vi "Prepend LBCB Number.vi"(1 "Prepended In":string[](array[string]), 2 "LBCB Number":T1, 3 "Names In":string[](array[string])) -> (0 "Prepended Out":string[](array[string]))   [LabVIEW 2013]
uses:
  Data Access Objects/Metadata/LBCB Number.ctl
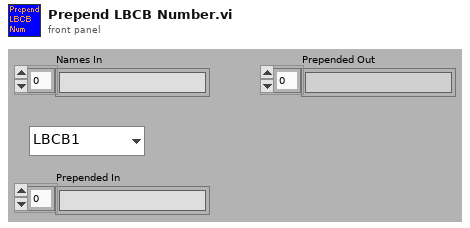
[diagram p1: front panel]
types:
  T1 = typedef "LBCB Number.ctl" = enum16{"LBCB1", "LBCB2"}
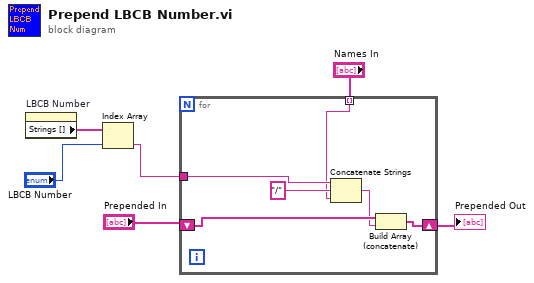
[diagram p0: block diagram]
diagram:
  n1 = property on="LBCB Number" class="Enum (strict)"() -> ("Strings []"=w3:string[])  [unwired: 2 in, 2 out]
  n2 = Index Array(array=w3, index="LBCB Number") -> (element=w1:string)
  n3 = for {
    shift-right: [w12] -> w6
    shift-left: "Prepended In" -> [w8]
    tunnel: w1 -> [w10]
    tunnel: "Names In" -> [w9] mode=indexing
    n4 = Concatenate Strings(w10, "/" ("string"), w9) -> (w7:string)
    n5 = Build Array (concatenate)(w8, w7) -> (w12:string[])
  }
  "Prepended Out" <- w6
